vi "mightexLiveview.vi"(11 "Close":bool) -> ()   [LabVIEW 2016]
uses:
  lib/SSClassic_USBCamera_SDK.dll
panel:
  in  "sharp":i32 min=0 max=3
  in  "bright":i32=50 min=0 max=100
  in  "contrast":i32=50 min=0 max=100
  in  "gamma":i32=10 min=1 max=20
  in  "Gain?":bool
  in  "Blue Gain":i32(slide)=17 scale=1.0..64.0
  in  "Green Gain":i32(slide)=16 scale=1.0..64.0
  in  "Red Gain":i32(slide)=20 scale=1.0..64.0
  out "new picture":picture
  out "ET Labelµ":dbl format="%#_3g"
  in  "Exposure Time:":dbl(slide) scale=1.0..100.0
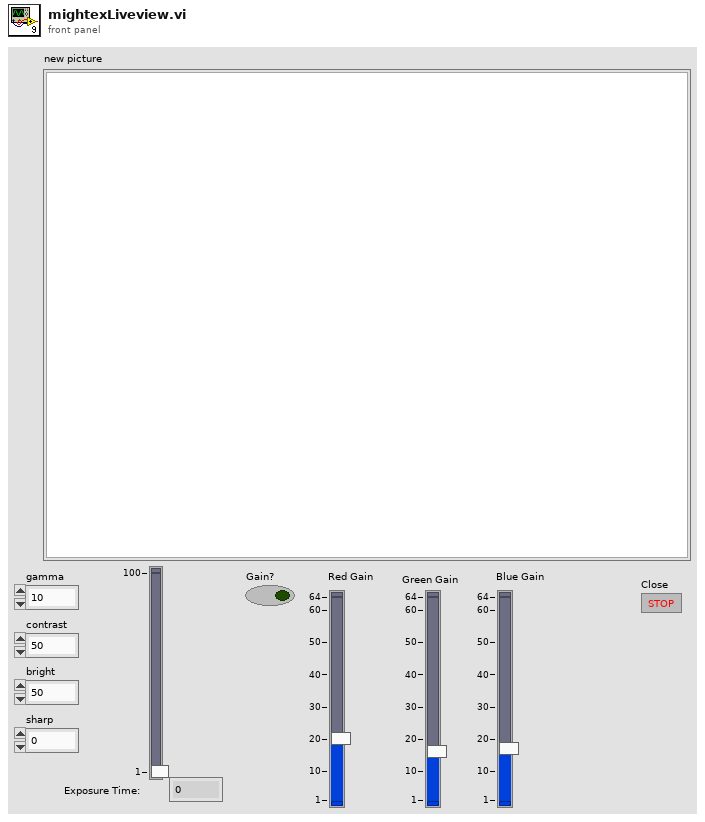
[diagram p1: front panel]
types:
  T1 = typedef "imagedata.ctl" = cluster{"image type":i32, "image depth":i32, "image":u8[], "mask":u8[], "colors":u32[], "Rectangle":cluster{"left":i16, "top":i16, "right":i16, "bottom":i16}}
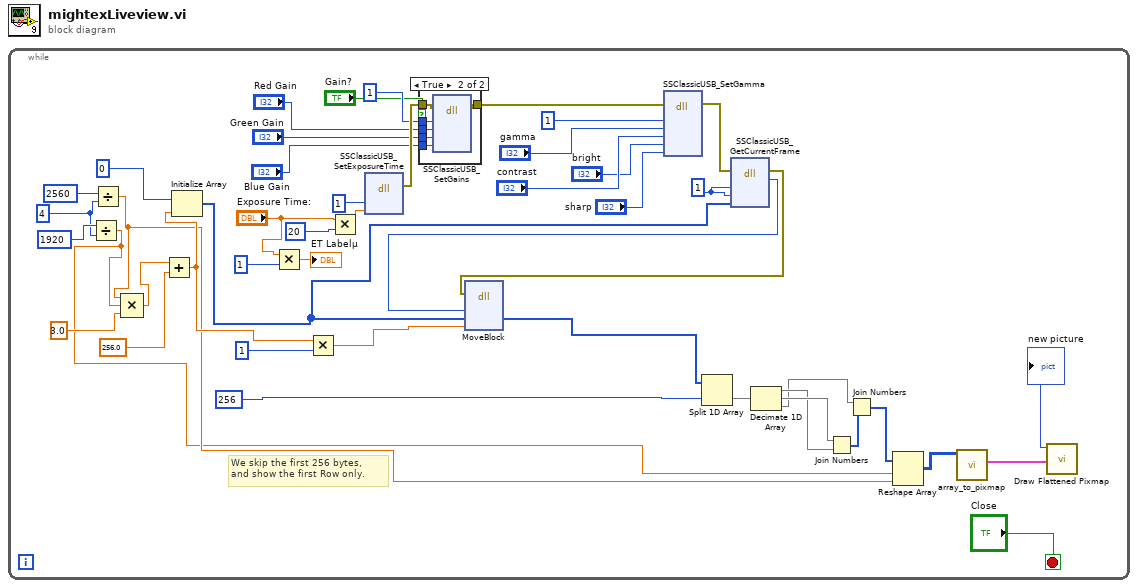
[diagram p0: block diagram]
diagram:
  n1 = while {
    stop <- "Close" stop-if-true
    w8 = 4 ("y")
    w37 = 1
    # "We skip the first 256 bytes,\nand show the first Row only."
    n2 = Divide(x=1920, y=w8) -> (x/y=w1:dbl)
    n3 = Divide(x=2560, y=w8) -> (x/y=w2:dbl)
    n4 = Compound Arithmetic op=MULTIPLY(w2, w1, 3.0 ("y")) -> (w3:dbl)
    n5 = Add(x=w3, y=256.0) -> (x+y=w5:dbl)
    n6 = Initialize Array(u8 0, w5) -> (w6:u8[])
    n7 = Multiply(x="Exposure Time:", y=1) -> (x*y=→"ET Labelµ":dbl)
    n8 = Multiply(x=w5, y=1) -> (x*y=w38:dbl)
    n9 = Multiply(x="Exposure Time:", y=20) -> (x*y=w42:dbl)
    n10 = dll-call lib="D:/All users/PoSheng/src/lib/SSClassic_USBCamera_SDK.dll" fn="SSClassicUSB_SetExposureTime" ("CCD_USBCamera_SDK.dll:CCDUSB_SetExposureTime")("Arg1"=1, "Arg2"=w42) -> (error out=w25:errorcluster)  [unwired: 6 in, 1 out]
    n11 = case shown="True" "Gain?" {
      tunnel: w25 -> [w48 w54]
      tunnel: [w48 w53] -> w18
      tunnel: 1 ("deviceID") -> [_ w52]
      tunnel: "Red Gain" -> [_ w51]
      tunnel: "Green Gain" -> [_ w50]
      tunnel: "Blue Gain" -> [_ w49]
      frame False {
      }
      frame True {
        n12 = dll-call lib="D:/All users/PoSheng/src/lib/SSClassic_USBCamera_SDK.dll" fn="SSClassicUSB_SetGains" ("CCD_USBCamera_SDK.dll:CCDUSB_SetExposureTime")(error in=w54, "deviceID"=w52, "redGain"=w51, "greenGain"=w50, "blueGain"=w49) -> (error out=w53:errorcluster)  [unwired: 7 in, 1 out]
      }
    }
    n13 = dll-call lib="D:/All users/PoSheng/src/lib/SSClassic_USBCamera_SDK.dll" fn="SSClassicUSB_SetGamma" ("CCD_USBCamera_SDK.dll:CCDUSB_GetCurrentFrame")(error in=w18, "deviceID"=1, "gamma"="gamma", "contrast"="contrast", "bright"="bright", "sharp"="sharp") -> (error out=w17:errorcluster)  [unwired: 8 in, 1 out]
    n14 = dll-call lib="D:/All users/PoSheng/src/lib/SSClassic_USBCamera_SDK.dll" fn="SSClassicUSB_GetCurrentFrame" ("CCD_USBCamera_SDK.dll:CCDUSB_GetCurrentFrame")(error in=w17, "Arg1"=w37, "Arg2"=w37, "Arg3"=w6) -> (error out=w26:errorcluster, "ReturnValue"=w46:i64)  [unwired: 5 in, 1 out]
    n15 = dll-call lib="LabVIEW" fn="MoveBlock"(error in=w26, "src"=w46, "dst"=w6, "size"=w38) -> ("dst"=w31:u8[])  [unwired: 5 in, 2 out]
    n16 = Split 1D Array(array=w31, index=256 ("y")) -> (second subarray=w36:u8[])  [unwired: 1 out]
    n17 = Decimate 1D Array(w36) -> (w33:u8[], w34:u8[], w27:u8[])
    n18 = Join Numbers(hi=w34, lo=w33) -> ((hi.lo)=w35:u16[])
    n19 = Join Numbers(hi=w27, lo=w35) -> ((hi.lo)=w32:u32[])
    n20 = Reshape Array(w32, w1, w2) -> (w30:u32[][])
    n21 = call "array_to_pixmap.vi"("photoarray"=w30) -> ("pixmap out"=w29:T1)  [unwired: 9 in, 1 out]
    n22 = call <vilib>:"Draw Flattened Pixmap.vi"("image data"=w29) -> ("new picture"=→"new picture":picture)  [unwired: 8 in]
  }
